vi "GE 5565PIORC.Memory.Write to DMA Block.vi"   [LabVIEW 2016, in "GE 5565PIORC.lvclass"]
doc: "Writes the contents of the <B>data</B> array to the specified <B>Block Descriptor</B>. The number of elements transferred will be either the number of elements in <B>data</B> or a number of elements resulting in a size that is less than or equal to the allocated size of the <B>Block Descriptor</B>, whichever is smaller."
uses:
  GE 5565PIORC.lvclass
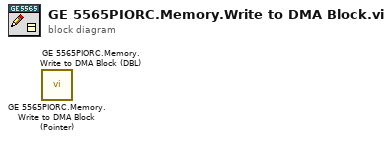
[diagram p0: block diagram]
diagram:
  n1 = call "GE 5565PIORC.Memory.Write to DMA Block (Pointer).vi"() -> ()  [unwired: 8 in, 4 out]
  n2 = call "GE 5565PIORC.Memory.Write to DMA Block (DBL).vi"() -> ()  [unwired: 8 in, 4 out]
